vi "Get Parent Actor Starting Folder Path.vi"(8 "error in (no error)":errorcluster) -> (0 "error out":errorcluster, 3 "Path String":path)   [LabVIEW 2023, in "Add Actor.lvlib"]
uses:
  Add Actor.lvlib
  <resource>/dialog/lvconfig.llb/LV Config Read Pathlist.vi
  AFPP Shared/AFPP Shared.lvlib
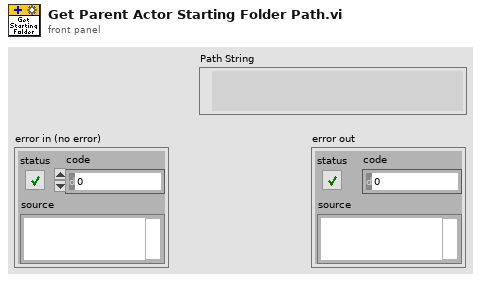
[diagram p1: front panel]
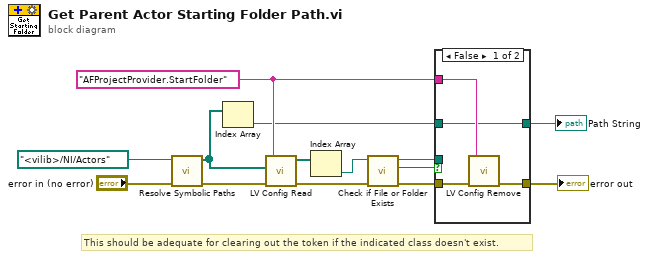
[diagram p0: block diagram]
diagram:
  w9 = "AFProjectProvider.StartFolder" ("key")
  # "This should be adequate for clearing out the token if the indicated class doesn't exist."
  n1 = call "Resolve Symbolic Paths.vi"("error in (no error)"="error in (no error)", "Path"=path "<vilib>/NI/Actors") -> ("error out"=w1:errorcluster, "Resolved Paths"=w4:path[])  [unwired: 8 in]
  n2 = Index Array(array=w4) -> (element=w5:path)  [unwired: 1 in]
  n3 = call-poly <resource>:"LV Config Read.vi"("error in"=w1, "default value"=w4, "key"=w9) -> ("error out"=w12:errorcluster, "value"=w14:path[])  [unwired: 2 in, 1 out]
  n4 = Index Array(array=w14) -> (element=w13:path)  [unwired: 1 in]
  n5 = call <vilib>:"Check if File or Folder Exists.vi"("error in (no error)"=w12, "path"=w13) -> ("error out"=w11:errorcluster, "file or folder exists?"=w8:bool, "dup path"=w6:path)  [unwired: 7 in]
  n6 = case shown="False" w8 {
    tunnel: w11 -> [w18 w20]
    tunnel: [w17 w20] -> w10
    tunnel: w9 -> [w16 _]
    tunnel: w5 -> [w15 _]
    tunnel: [w15 w19] -> w7
    tunnel: w6 -> [_ w19]
    frame False {
      n7 = call <resource>:"LV Config Remove.vi"("error in"=w18, "key"=w16) -> ("error out"=w17:errorcluster)  [unwired: 5 in]
    }
    frame True {
    }
  }
  "error out" <- w10
  "Path String" <- w7
